vi "A Auto Aim.vi"() -> ()   [LabVIEW 2015]
uses:
  Robot Global Data.vi
panel:
  out "Potentiometer":dbl
  out "Dart Length(in)":dbl
  out "Angle":dbl
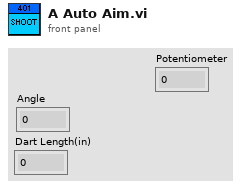
[diagram p1: front panel]
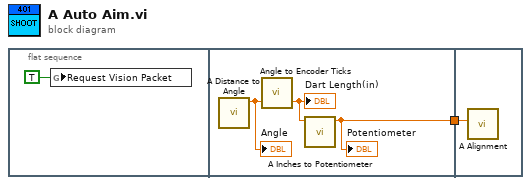
[diagram p0: block diagram]
diagram:
  n1 = flat-sequence {
    tunnel: [w5] -> w1
    tunnel: w1 -> [w6]
    frame #0 {
      n2 = global write "Robot Global Data.vi" "Request Vision Packet"(TRUE) -> ()
    }
    frame #1 {
      n3 = call "A Distance to Angle.vi"() -> ("Angle"=w4:dbl)  [unwired: 11 in]
      "Angle" <- w4
      n4 = call "Angle to Encoder Ticks.vi"("Angle(degrees)"=w4) -> ("Dart Length(in)"=w3:dbl)  [unwired: 1 in, 1 out]
      "Dart Length(in)" <- w3
      n5 = call "A Inches to Potentiometer.vi"("Inches"=w3) -> ("Potentiometer"=w5:dbl)  [unwired: 10 in]
      "Potentiometer" <- w5
    }
    frame #2 {
      n6 = call "A Alignment.vi"("Potentiometer Value"=w6) -> ()  [unwired: 11 in]
    }
  }
